vi "Monitor for Stop.vi"(8 "error in (no error)":errorcluster, 9 "Mixed Mode Commands In":refnum<queue>, 11 "MM Button Events In":refnum<notifier>) -> (0 "error out":errorcluster, 1 "Mixed Mode Commands Out":refnum<queue>, 3 "Button Events Out":refnum<notifier>)   [LabVIEW 2009]
uses:
  Mixed Mode Button Events Message.ctl
  Mixed Mode Button Events.ctl
  Mixed Mode Widget Button States.ctl
  Mixed Mode Control Type.ctl
  Messages/Mixed Mode Command.ctl
  Mixed Mode Command Action.ctl
  Ramp Time Tuple.ctl
  Target Data.ctl
  Data Access Objects/Metadata/LBCB Space.ctl
panel:
  out "Stop Requested":bool
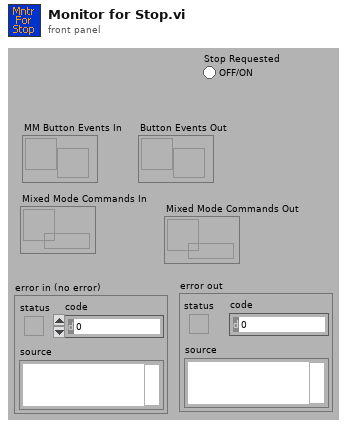
[diagram p1: front panel]
types:
  T1 = typedef "Mixed Mode Command.ctl" = cluster{"Command":T2, "Ramp Times":cluster{"Initial":T3, "Iterative":T3}, "LBCB1":T4, "LBCB2":T4}
  T2 = typedef "Mixed Mode Command Action.ctl" = enum16{"Start Command", "Stop", "Exit", "No Op", "Start Acquisition", "Measure Initial Position"}
  T3 = typedef "Ramp Time Tuple.ctl" = cluster{"Ramp":dbl, "Stab":dbl, "Hold":dbl}
  T4 = typedef "Target Data.ctl" = cluster{"Displacements":dbl[], "Command Type":enum16{"<None>", "Displacement", "Force"}[], "Forces":dbl[], "Space":T5}
  T5 = typedef "LBCB Space.ctl" = enum16{"Actuator", "Cartesian"}
  T6 = typedef "Mixed Mode Button Events Message.ctl" = cluster{"MM Control Events":T7, "Button States":T8}
  T7 = typedef "Mixed Mode Button Events.ctl" = enum16{"Propose.Accept", "Propose.Decline", "Execute.Start", "Execute.Stop", "TargetChange", "InputFile.Load", "InputFile.Reset", "InputFile.Pause", "InputFile.Run", "CartesianType.Changed", "NCTP.ConnectToServer", "Application.Stop", "Control.Enabled", "Control.Disabled", "ControlType.Changed", "Nop"}
  T8 = typedef "Mixed Mode Widget Button States.ctl" = cluster{"Auto-Start Enabled":bool, "Auto-Accept Enabled":bool, "Exit Requested":bool, "Mixed Mode Control Type":T9, "Input File Loaded":bool, "Input File Running":bool}
  T9 = typedef "Mixed Mode Control Type.ctl" = enum32{"Manual", "Input File", "NTCP"}
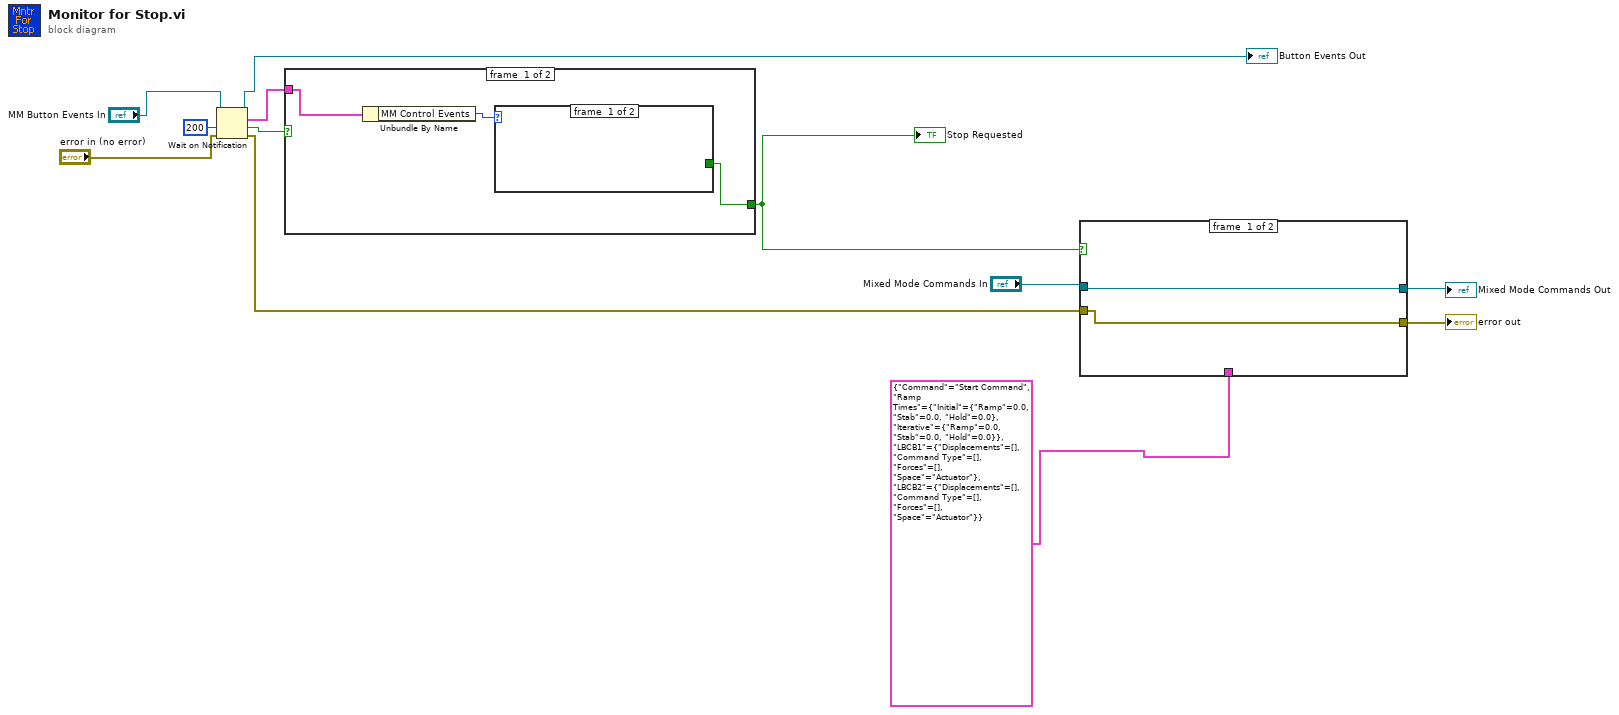
[diagram p0: block diagram]
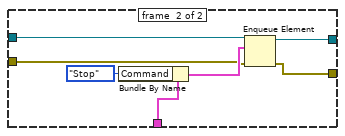
[diagram p2: hidden frame]
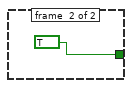
[diagram p3: hidden frame]
diagram:
  n1 = Wait on Notification(notifier="MM Button Events In", timeout in ms (-1)=200, error in (no error)="error in (no error)") -> (notifier out=→"Button Events Out":refnum<notifier>, notification=w7:T6, timed out?=w8:bool, error out=w5:errorcluster)  [unwired: 1 in]
  n2 = case shown="False" w8 {
    tunnel: w7 -> [w15 _]
    tunnel: [w13 _] -> w1
    frame #0 {
      n3 = Unbundle By Name(w15) -> ("MM Control Events"=w14:T7)
      n4 = case shown="\"Execute.Stop\"" w14 {
        tunnel: [_ TRUE] -> w13
        frame #0 {
        }
        frame #1 {
        }
      }
    }
    frame #1 {
    }
  }
  "Stop Requested" <- w1
  n5 = case shown="True" w1 {
    tunnel: "Mixed Mode Commands In" -> [w17 w25]
    tunnel: T1 {"Command"=enum."Start Command", "Ramp Times"={"Initial"={"Ramp"=0.0, "Stab"=0.0, "Hold"=0.0}, "Iterative"={"Ramp"=0.0, "Stab"=0.0, "Hold"=0.0}}, "LBCB1"={"Displacements"=[], "Command Type"=[], "Forces"=[], "Space"=enum."Actuator"}, "LBCB2"={"Displacements"=[], "Command Type"=[], "Forces"=[], "Space"=enum."Actuator"}} ("Mixed Mode Command") -> [_ w24]
    tunnel: [w17 w22] -> w2
    tunnel: [w18 w21] -> w6
    tunnel: w5 -> [w18 w20]
    frame #0 {
    }
    frame #1 {
      n6 = Bundle By Name(cluster=w24, "Command"=Mixed_Mode_Command_Action."Stop") -> (w23:T1)
      n7 = Enqueue Element(queue=w25, element=w23, error in (no error)=w20) -> (queue out=w22:refnum<queue>, error out=w21:errorcluster)  [unwired: 1 in, 1 out]
    }
  }
  "error out" <- w6
  "Mixed Mode Commands Out" <- w2
